vi "nPoints Concept - LED.vi"() -> ()   [LabVIEW 2013]
uses:
  <vilib>/DAQmx/write.llb/DAQmx Write (Digital 1D Bool 1Chan 1Samp).vi
  <vilib>/DAQmx/create/channels.llb/DAQmx Create Channel (DO-Digital Output).vi
  <vilib>/DAQmx/miscellaneous.llb/DAQmx Fill In Error Info.vi
panel:
  out "Waveform Chart":cluster{"[0]":i16, "[1]":i16, "[2]":i16}(graph)
  in  "Blink Time (ms)":u32=500
  in  "Blink":bool
  in  "Yellow LED":bool
  in  "Green LED":bool
  in  "Red LED":bool
  in  "Stop":bool
  # "Light Emitting Diode"
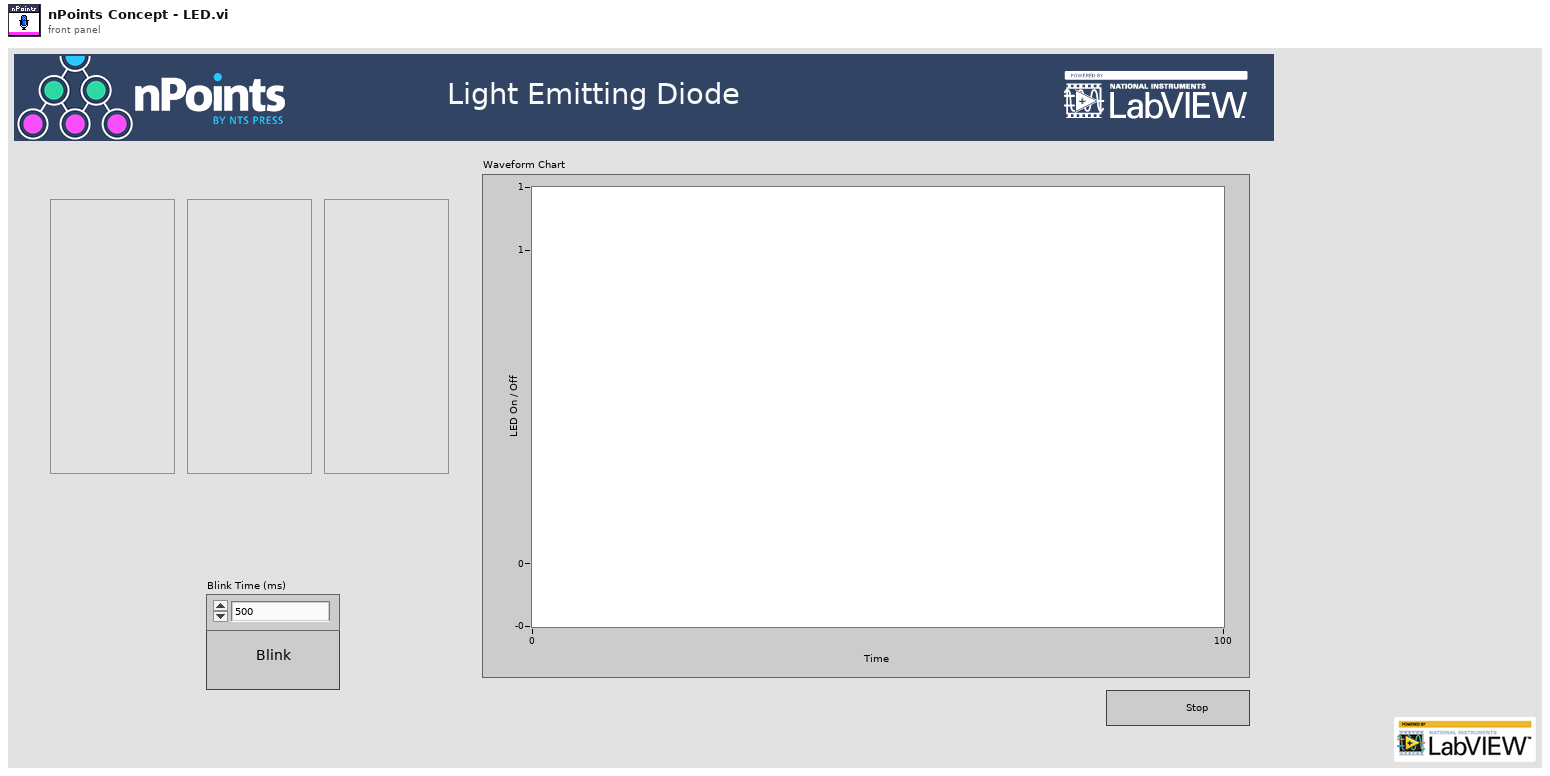
[diagram p1: front panel]
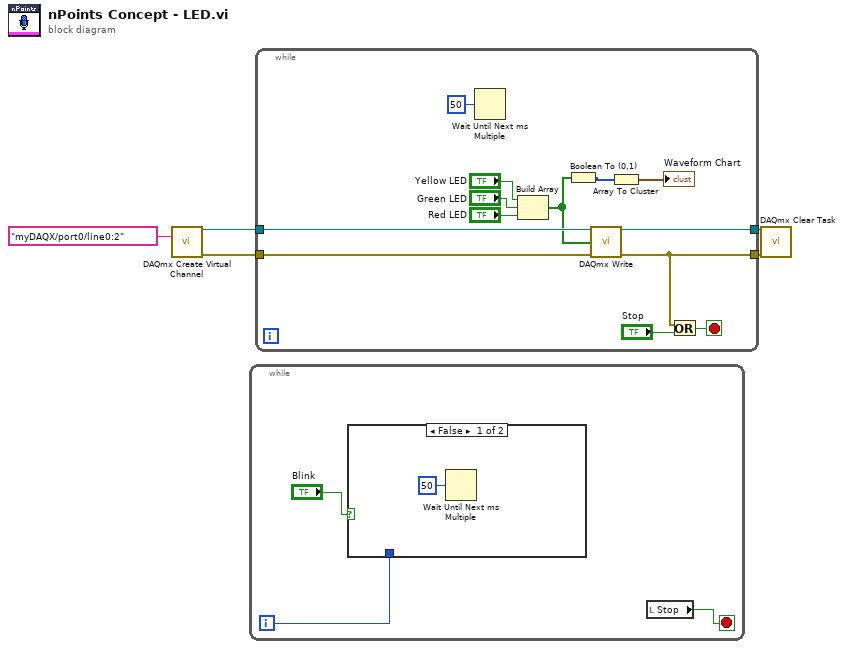
[diagram p0: block diagram]
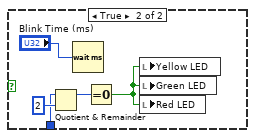
[diagram p2: hidden frame]
diagram:
  n1 = call-poly <vilib>:"DAQmx Create Virtual Channel.vi"("lines"=tag "myDAQX/port0/line0:2") -> ("task out"=w1:refnum<k21>, "error out"=w3:errorcluster)  [unwired: 13 in]
  n2 = while {
    i -> [w8]
    stop <- w7 stop-if-true
    n3 = case shown="False" "Blink" {
      tunnel: w8 -> [_ w10]
      frame False {
        n4 = Wait Until Next ms Multiple(millisecond multiple=u32 50) -> ()  [unwired: 1 out]
      }
      frame True {
        n5 = Quotient & Remainder(x=w10, y=2) -> (x-y*floor(x/y)=w12:i32)  [unwired: 1 out]
        n6 = Wait (ms)(milliseconds to wait="Blink Time (ms)") -> ()  [unwired: 1 out]
        n7 = Equal To 0?(x=w12) -> (x = 0?=w11:bool)
        n8 = local write "Yellow LED"(w11) -> ()
        n9 = local write "Green LED"(w11) -> ()
        n10 = local write "Red LED"(w11) -> ()
      }
    }
    n11 = local read "Stop"() -> (w7:bool)
  }
  n12 = while {
    tunnel: w3 -> [w24]
    tunnel: w1 -> [w25]
    tunnel: [w23] -> w5
    tunnel: [w22] -> w4
    stop <- w26 stop-if-true
    n13 = Wait Until Next ms Multiple(millisecond multiple=u32 50) -> ()  [unwired: 1 out]
    n14 = Build Array("Yellow LED", "Green LED", "Red LED") -> (w17:bool[])
    n15 = Boolean To (0,1)(Boolean=w17) -> (0, 1=w16:i16[])
    n16 = call-poly <vilib>:"DAQmx Write.vi"("task/channels in"=w25, "data"=w17, "error in"=w24) -> ("task out"=w23:refnum<k21>, "error out"=w22:errorcluster)  [unwired: 10 in, 1 out]
    n17 = Array To Cluster(array=w16) -> (cluster=→"Waveform Chart":cluster{"[0]":i16, "[1]":i16, "[2]":i16})
    n18 = Or(x=w22, y="Stop") -> (x .or. y?=w26:bool)
  }
  n19 = call <vilib>:"DAQmx Clear Task.vi"("task in"=w5, "error in"=w4) -> ()  [unwired: 13 in, 1 out]
